vi "Main.vi"() -> ()   [LabVIEW 2013]
doc: "This template is for the Queued Message Handler design pattern.\n\nThe Event Handling Loop generates messages based on user interface actions.\n\nThe Message Handling Loop processes messages generated by the Event Handling Loop, or by other messages. The messages are string values, so new messages can be added easily to the Message Cases case structure in the Message Handling Loop. Each message cluster can also provide an optional value for Message Data, which is a variant that can be converted to whatever message-specific data is required."
uses:
  <vilib>/vision/Image Controls.llb/IMAQ Image.ctl
  Message Passing/MsgQ Loops enum.ctl
  Image Processing/Mask ROI FG Enum.ctl
  System Status/Status FG Enum.ctl
  Globals/Average Sector Data.vi
  controls/UI Data.ctl
  Message Queue/Message Queue.lvlib
  User Event - Stop/User Event - Stop.lvlib
  Image Processing/Image Processing.lvlib
  Common/State Machines/State Machine Lib.lvlib
  Message Passing/Main MsgQ.lvlib
  Common/GUI/GUI.lvlib
panel:
  out "Log Start (s)":dbl caption="Present (s)"
  in  "minutes to log":dbl=22.0
  out "Acq FIFO Timeout":bool
  out "Host DMA Timeout":bool
  in  "Log?":bool
  out "Log Input Signal":bool
  out "# of extracted frames":u32=1
  in  "Update Display?":bool=TRUE
  out "write time":dbl
  out "Frame Count":u16=1
  out "Frames Acquired":u32=11578
  in  "Disable Background Subtraction":bool
  out "FPGA Display Image":T1(plugin-control)
  out "Right Wingbeat Avg Graph":u8[](graph)=[71, 91, 86, 73, 55, 38, 22, 8, 3, 0, 0, 0, 0, 0, 0, 0]
  in  "Start Serial Server":bool=TRUE
  out "Left Wingbeat Avg Graph":u8[](graph)=[106, 114, 100, 76, 51, 28, 9, 0, 0, 0, 0, 0, 0, 0, 0, 0]
  in  "Stop Charts":bool
  in  "Wing ROIs":T2
  out "FPGA image info":T5={"Image Type"=0, "Unit"=enum."Undefined", "X Resolution"=1200, "Y Resolution"=788, "X Step"=1.0, "Y Step"=1.0, "Image Name"="Acquired"} {"Image Type" items=["Grayscale (U8)", "Grayscale (I16)", "Grayscale (SGL)", "Complex (CSG)", "RGB (U32)", "HSL (U32)", "RGB (U64)", "Grayscale (U16)"]}
  in  "Stream?":bool
  out "FPGA Image":T1
  in  "Test Visual Response":bool
  in  "Test FPGA":bool
  out "Status Update":string="09/25/2015 16:02:54.861 :  Camera Initialized\r"
  in  "Define Mask":bool
  in  "Acquire Image":bool
  in  "Stop":bool
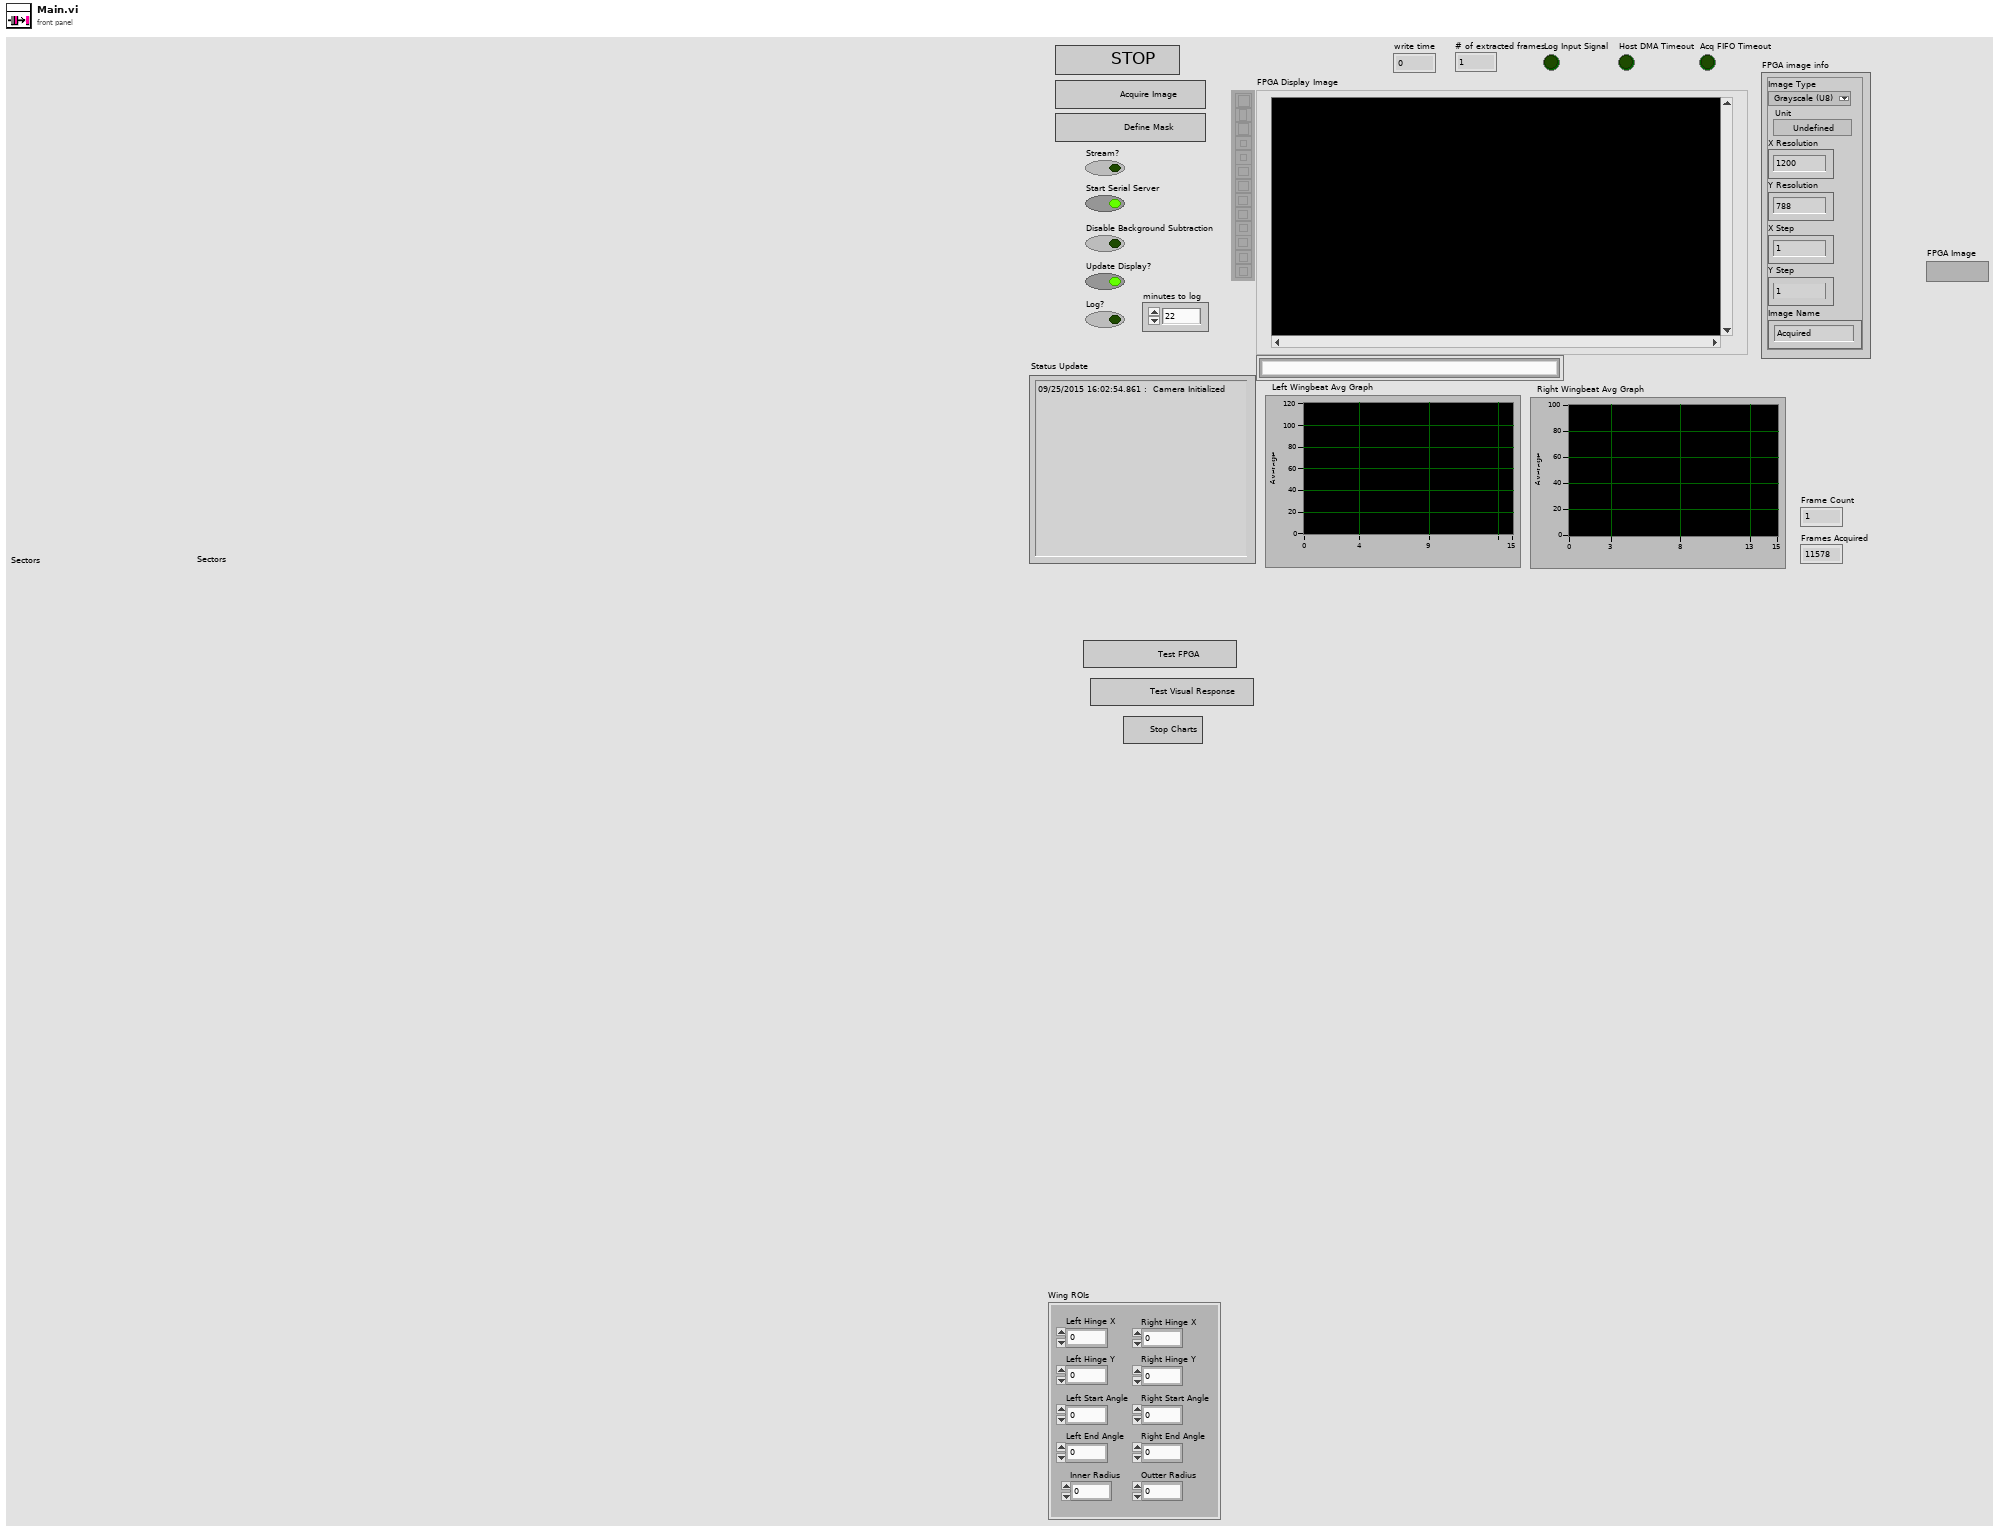
[diagram p1: front panel]
types:
  T1 = typedef "IMAQ Image.ctl" = refnum<image>
  T2 = cluster{"Left Hinge X":u16, "Left Hinge Y":u16, "Inner Radius":u16, "Outter Radius":u16, "Right Hinge X":u16, "Right Hinge Y":u16, "Right Start Angle":i16, "Right End Angle":i16, "Left Start Angle":i16, "Left End Angle":i16}
  T3 = typedef "Image Type" = u32
  T4 = typedef "Image Unit" = enum32{"Undefined", "Angström", "Micrometer", "Millimeter", "Centimeter", "Meter", "Kilometer", "Microinch", "Inch", "Feet", "Nautical miles", "Standard miles", "Steps"}
  T5 = cluster{"Image Type":T3, "Unit":T4, "X Resolution":i32, "Y Resolution":i32, "X Step":sgl, "Y Step":sgl, "Image Name":string}
  T6 = typedef "State Machine Lib.lvlib/STATE cluster.ctl" = cluster{"State":string, "Parameters":variant}
  T7 = typedef "Main MsgQ.lvlib/MsgQ Loops enum.ctl" = enum16{"User Interface", "Image Acq"}
  T8 = typedef "Mask ROI FG Enum.ctl" = enum16{"Read", "Write", "Enable Background", "Disable Background"}
  T9 = typedef "Status FG Enum.ctl" = enum16{"Reset", "Read", "Write"}
  T10 = typedef "Mask ROI Cluster.ctl" = cluster{"left annulus":T11, "right annulus":T11, "Threshold Range":cluster{"Lower value":dbl, "Upper value":dbl}, "[Avg BG]":u8[], "Number of Sectors":u8, "Left ROI":T12, "Right ROI":T12, "Left Start Angle Duty Cycle":fxp<+,8,0>, "Left End Angle Duty Cycle":fxp<+,8,0>, "Right End Angle Duty Cycle":fxp<+,8,0>, "Right Start Angle Duty Cycle":fxp<+,8,0>, "[Sector ROIs]":T12[], "Consecutive Sector Threshold":u8}
  T11 = typedef "IMAQ Circle" = cluster{"Center X":i32, "Center Y":i32, "Inner Radius":i32, "Outer Radius":i32, "Start Angle":dbl, "End Angle":dbl}
  T12 = typedef "ROI Descriptor" = cluster{"Global Rectangle":i32[], "Contours":cluster{"ID":enum32{"External", "Internal"}, "Type":u32, "Coordinates":i32[]}[]}
  T13 = typedef "UI Data.ctl" = cluster{"Boolean <Replace Me>":bool, "Initial Message":string, "Numeric <Replace Me>":dbl, "Acquire Image Ref":refnum<vi>, "Define Mask Ref":refnum<vi>, "Status Update Ref":refnum<vi>, "Stop Button Ref":refnum<vi>, "FPGA Image":T1, "Processed Image":T1, "Left Annulus":cluster{"Center X":i32, "Center Y":i32, "Inner Radius":i32, "Outer Radius":i32, "Start Angle":dbl, "End Angle":dbl}, "Right Annulus":cluster{"Center X":i32, "Center Y":i32, "Inner Radius":i32, "Outer Radius":i32, "Start Angle":dbl, "End Angle":dbl}}
  T14 = typedef "Message Queue.lvlib/All Message Queues.ctl" = cluster{"UI":refnum<queue>}
  T15 = cluster{"Center X":i32, "Center Y":i32, "Inner Radius":i32, "Outer Radius":i32, "Start Angle":dbl, "End Angle":dbl}
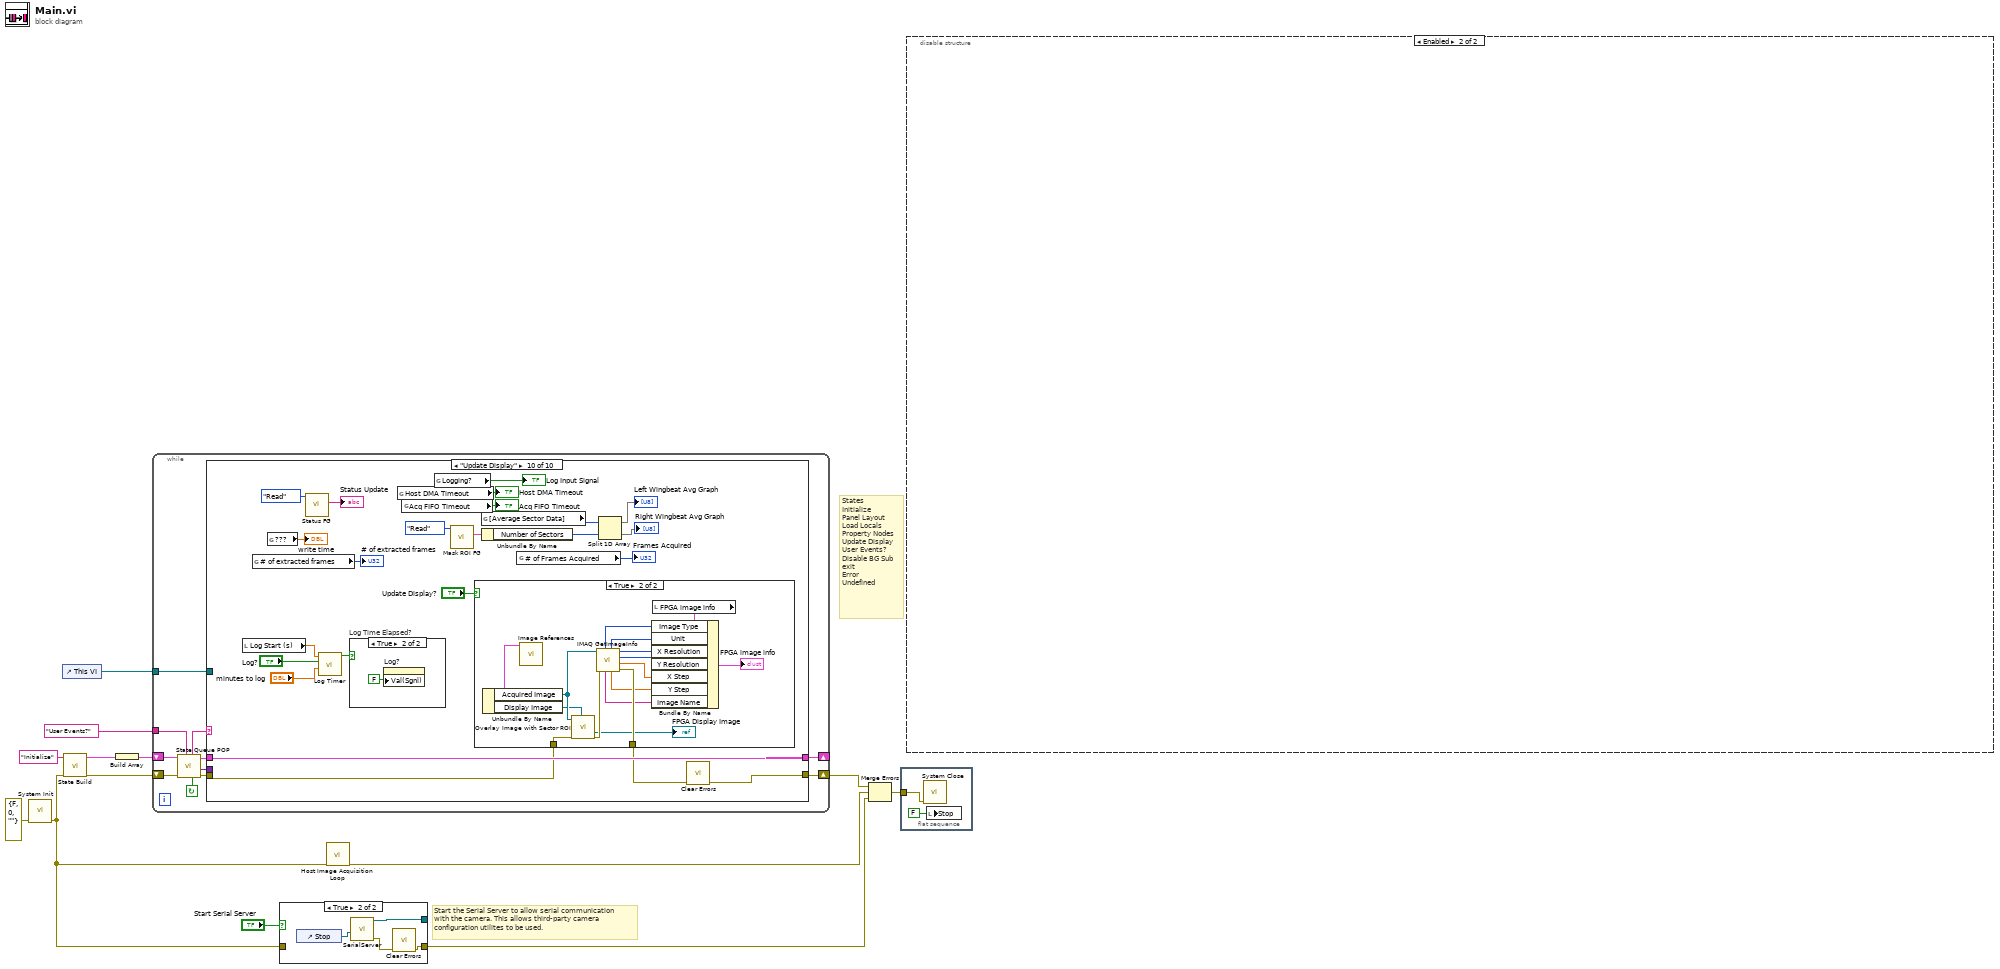
[diagram p0: block diagram]
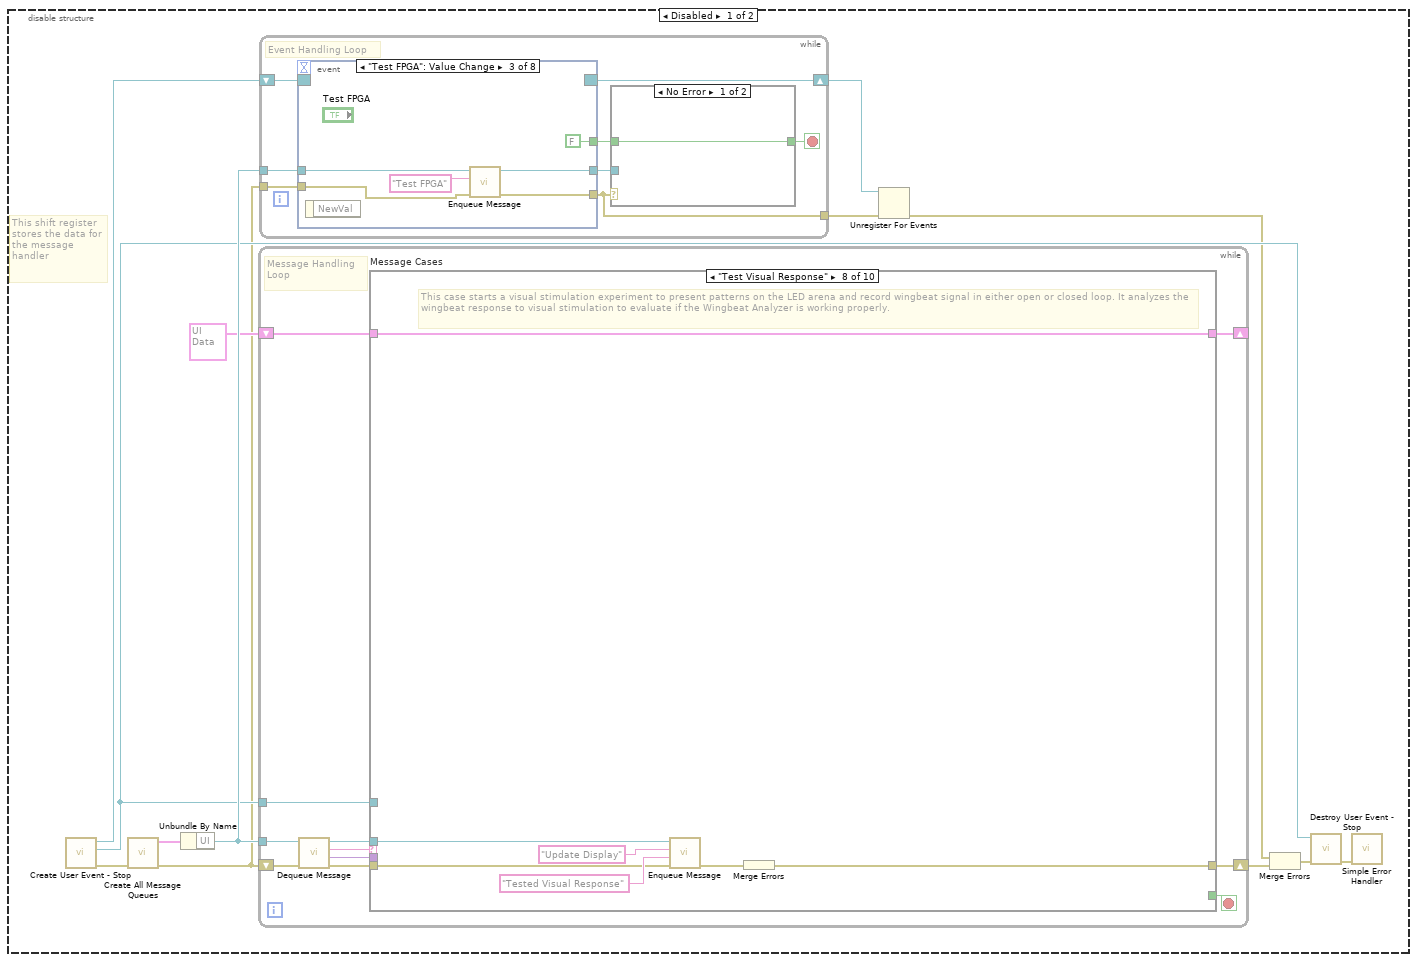
[diagram p3: hidden frame]
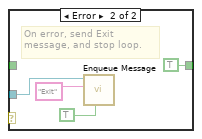
[diagram p4: hidden frame]
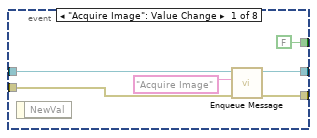
[diagram p5: hidden frame]
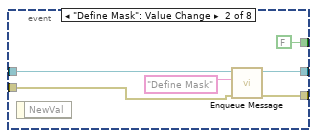
[diagram p6: hidden frame]
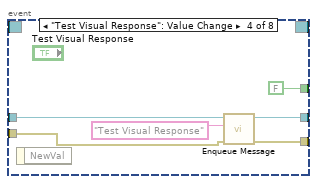
[diagram p7: hidden frame]
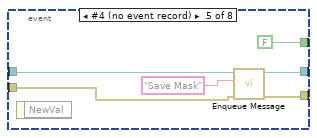
[diagram p8: hidden frame]
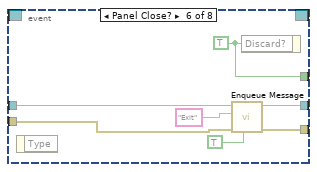
[diagram p9: hidden frame]
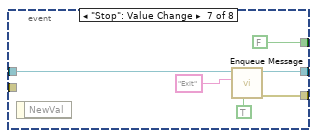
[diagram p10: hidden frame]
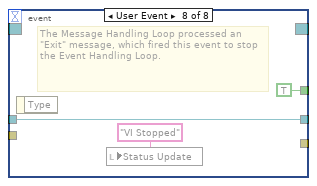
[diagram p11: hidden frame]
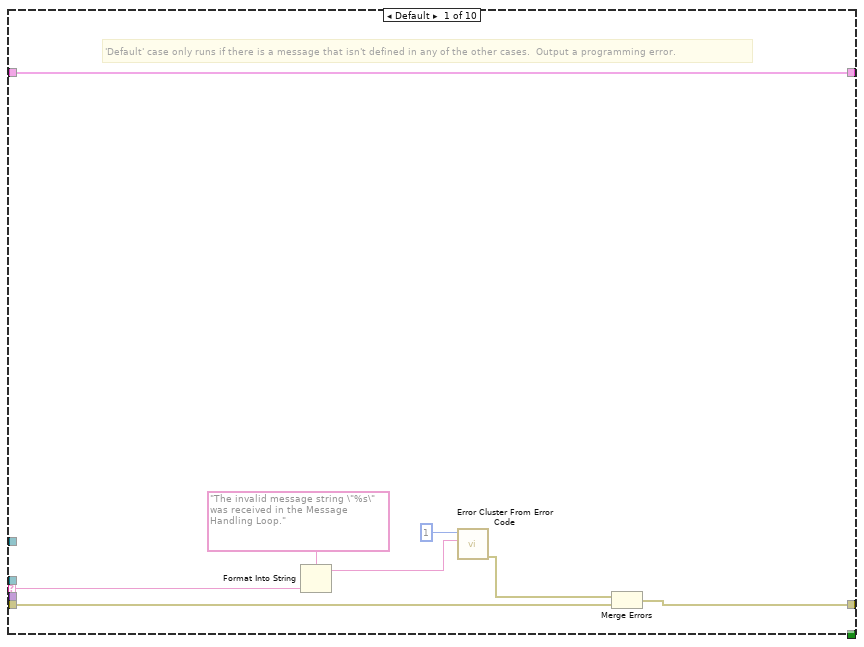
[diagram p12: hidden frame]
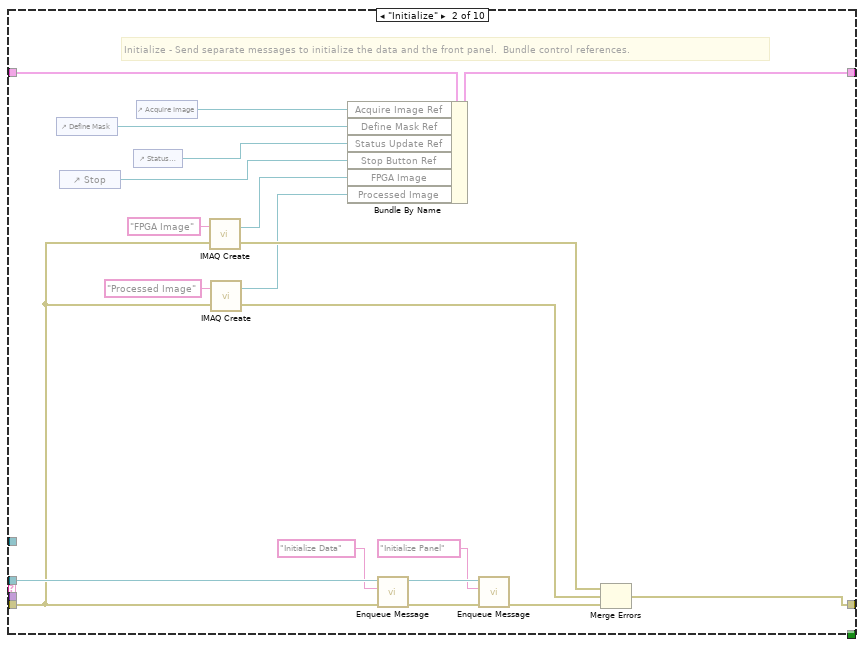
[diagram p13: hidden frame]
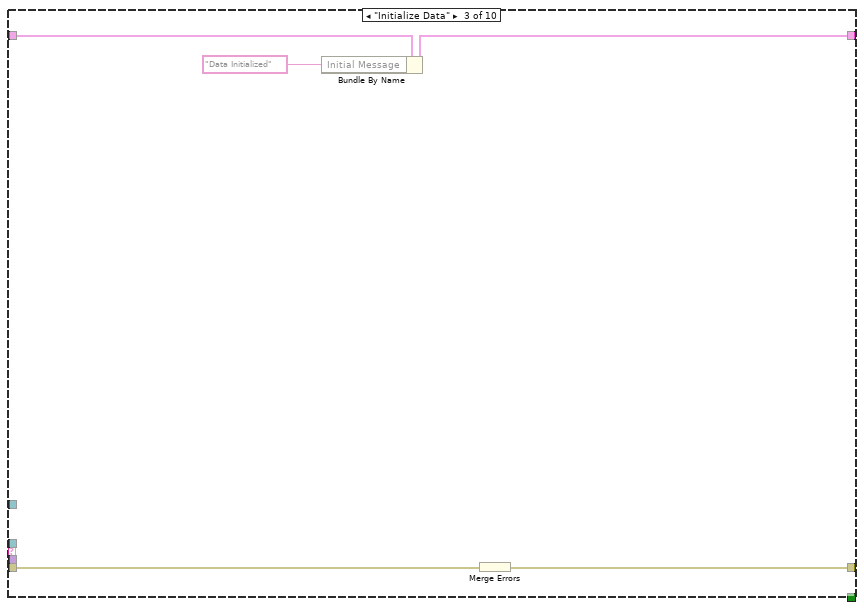
[diagram p14: hidden frame]
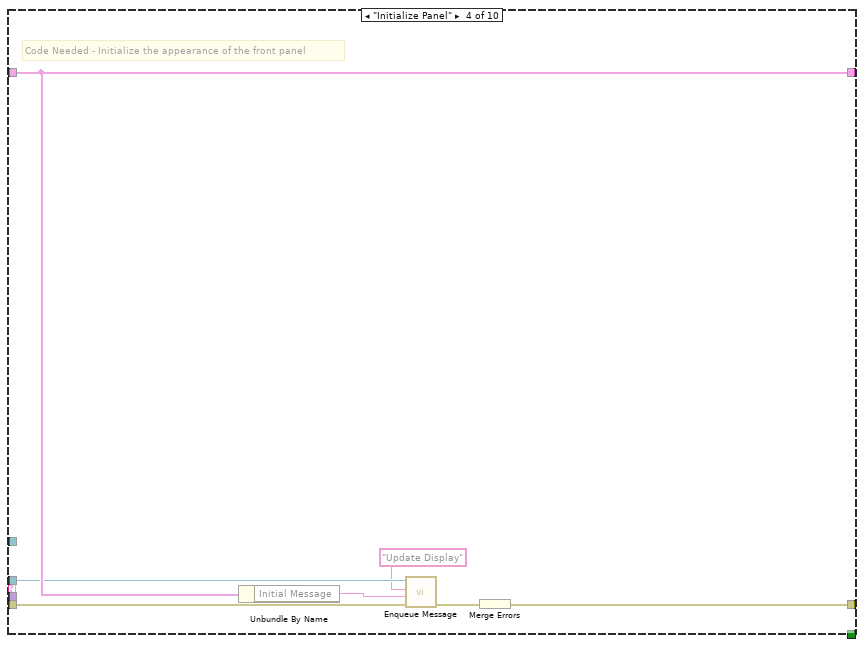
[diagram p15: hidden frame]
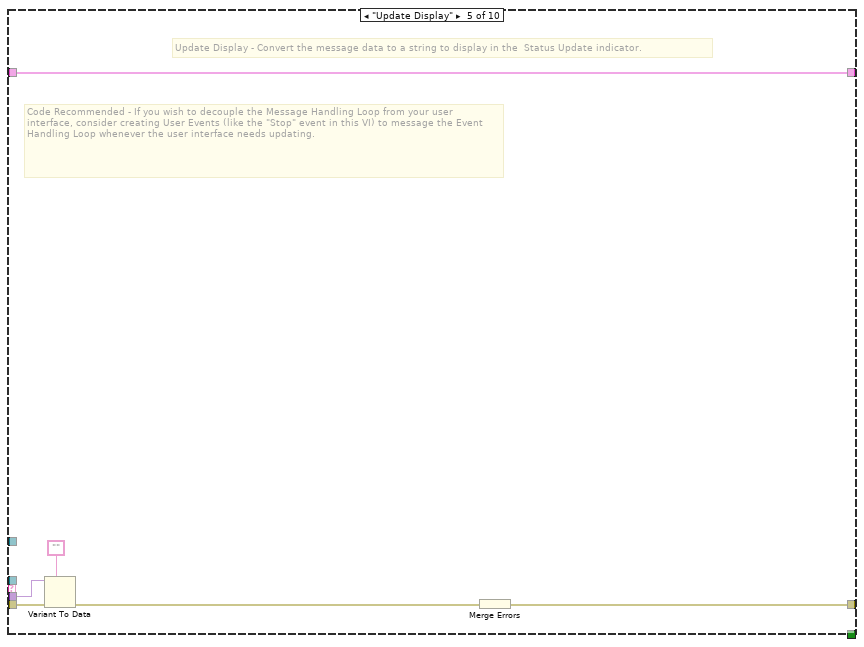
[diagram p16: hidden frame]
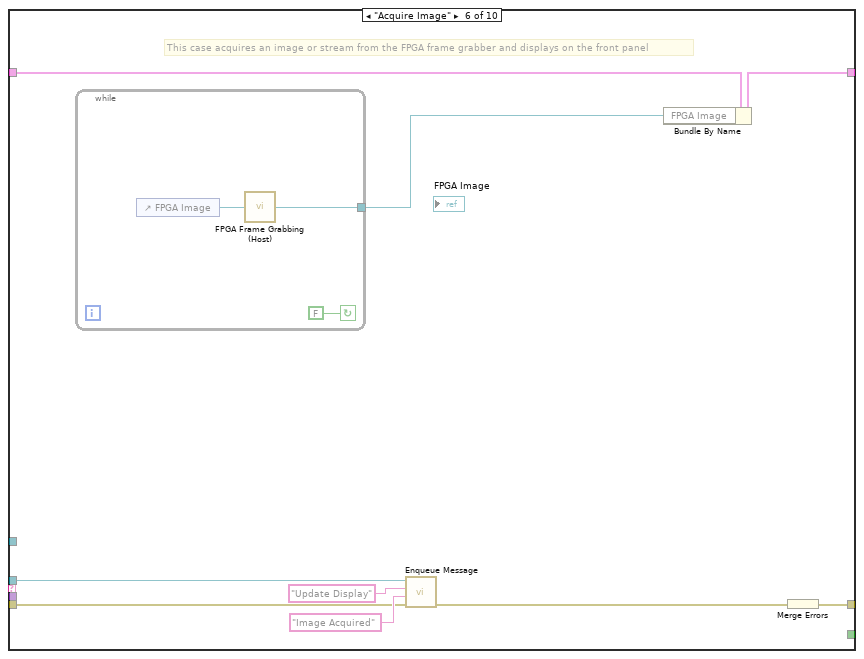
[diagram p17: hidden frame]
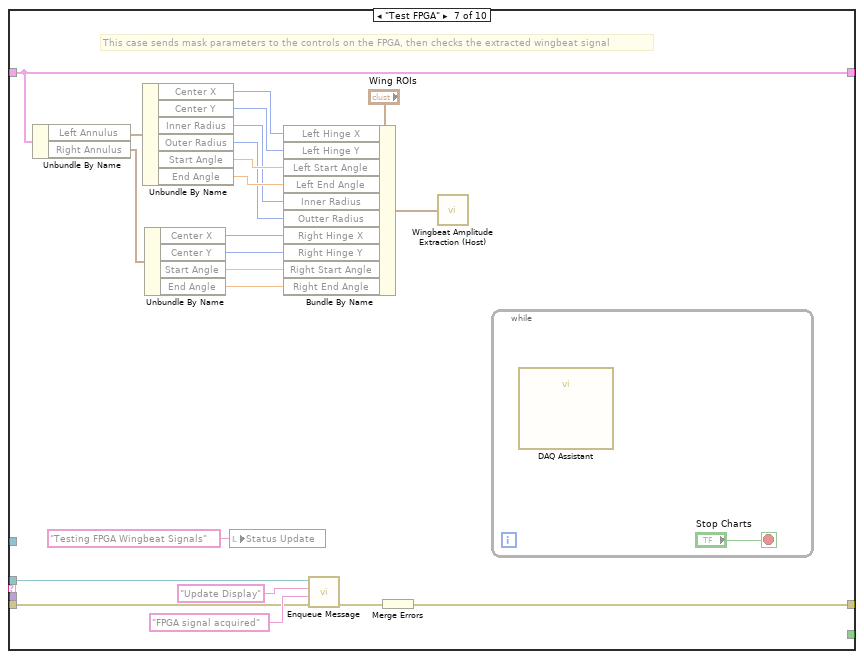
[diagram p18: hidden frame]
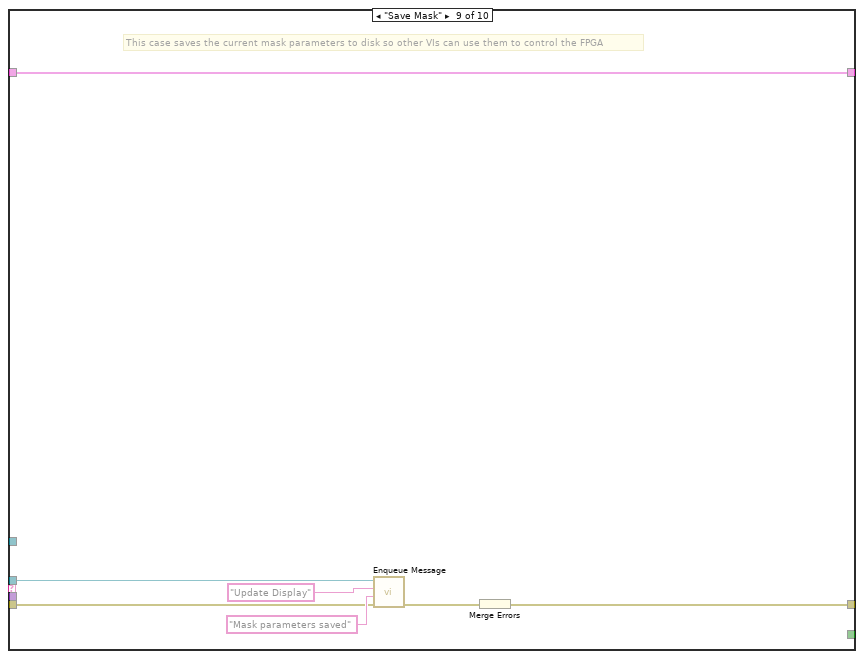
[diagram p19: hidden frame]
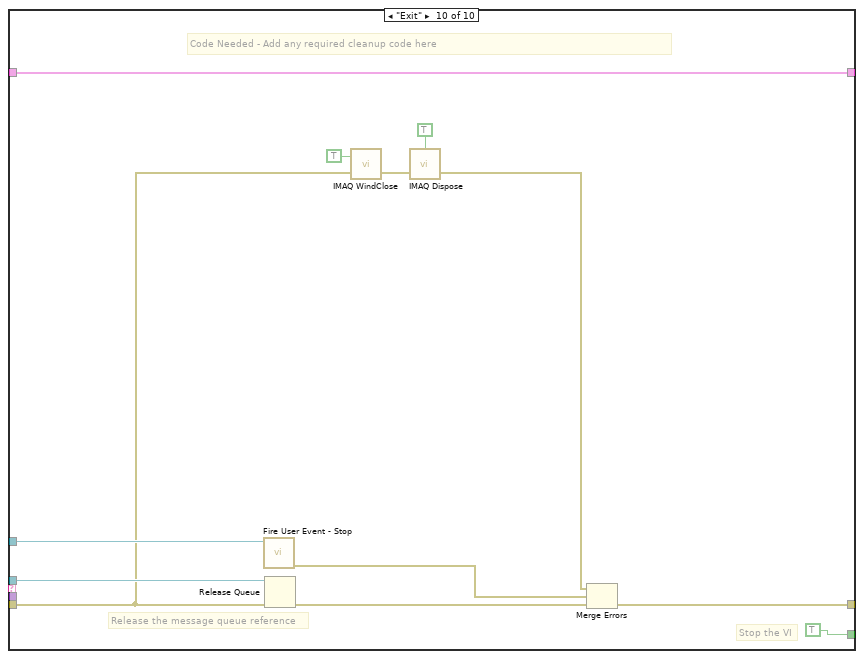
[diagram p20: hidden frame]
diagram:
  # "Start the Serial Server to allow serial communication\nwith the camera. This allows third-party camera\nconfiguration utilites to be used."
  # "States\nInitialize\nPanel Layout\nLoad Locals\nProperty Nodes\nUpdate Display\nUser Events?\nDisable BG Sub\nexit\nError\nUndefined"
  n1 = call "System Init.vi"("error in (no error)"=errorcluster {"status"=FALSE, "code"=0, "source"=""}) -> ("error out"=w12:errorcluster)  [unwired: 10 in]
  n2 = control-ref of="This VI"() -> (w6:refnum<vi>)
  n3 = call "State Build.vi"("error in (no error)"=w12, "State"="Initialize") -> ("error out"=w8:errorcluster, "State Out"=w10:T6)  [unwired: 8 in]
  n4 = Build Array(w10) -> (w9:T6[])
  n5 = while {
    shift-right: [w18] -> _
    shift-left: w9 -> [w24]
    shift-right: [w16] -> w5
    shift-left: w8 -> [w23]
    tunnel: "User Events?" ("State") -> [w21]
    tunnel: w6 -> [w19]
    stop <- w22 continue-if-true
    n6 = call "State Queue POP.vi"("Default state"=w21, "error in (no error)"=w23, "State que in"=w24) -> ("error out"=w15:errorcluster, "Parameters"=w14:variant, "State que out"=w17:T6[], "Not Exit?"=w22:bool, "State case out"=w20:string)  [unwired: 4 in]
    n7 = case shown="\"Update Display\"" w20 {
      tunnel: w19 -> [_ _ w35 _ _ _ _ _ _ _]
      tunnel: [w26 w27 w32 w41 w43 w48 w49 w66 w113 w137] -> w18
      tunnel: w17 -> [w26 w30 w32 w41 w43 w48 w49 w65 _ w137]
      tunnel: [w25 w28 w33 w36 w42 w46 w50 w64 w112 w136] -> w16
      tunnel: w15 -> [w25 w29 w34 w37 w42 w47 w61 w63 w114 w135]
      tunnel: w14 -> [_ _ _ _ _ _ w60 w62 _ _]
      frame Default {
      }
      frame "Initialize" {
        n8 = call "State Queue PUSH multiple states no parameters.vi"("States to queue"=string[] ["Panel Layout", "Load Locals", "Property Nodes", "Update Display"], "error in (no error)"=w29, "State que in"=w30) -> ("error out"=w28:errorcluster, "State que out"=w27:T6[])  [unwired: 7 in]
      }
      frame "Panel Layout" {
        # "Reset origin to 0,0"
        n9 = call "Reset all pane origins.vi"("error in (no error"=w34, "Vi Ref In"=w35) -> ("error out"=w33:errorcluster)  [unwired: 8 in, 1 out]
      }
      frame "Load Locals" {
        w40 = FALSE ("Stream?")
        n10 = call "Send MsgQ.vi"("error in (no error)"=w37, "Message String"="Close Save File" ("f"), "Send to MsgQ"=MsgQ_Loops_enum."Image Acq") -> ("error out"=w36:errorcluster)  [unwired: 8 in]
        n11 = local write "Stream?"(w40) -> ()
        n12 = local write "Disable Background Subtraction"(w40) -> ()
        n13 = local write "Log?"(w40) -> ()
      }
      frame "Property Nodes" {
      }
      frame "Define Mask" {
        n14 = call "Image References.vi"() -> ("Images"=w45:cluster{"Acquired Image":T1, "Display Image":T1})  [unwired: 10 in, 1 out]
        n15 = Unbundle By Name(w45) -> ("Acquired Image"=w44:T1)
        n16 = call "Define Mask.vi"("error in (no error)"=w47, "FPGA Image"=w44) -> ("error out"=w46:errorcluster)  [unwired: 9 in]
      }
      frame "Disable BG Sub" {
        n17 = Variant To Data(error in=w61, type=FALSE, Variant=w60) -> (data=w58:bool, error out=w55:errorcluster)
        n18 = Select(t=Mask_ROI_FG_Enum."Disable Background" ("Operation"), s=w58, f=Mask_ROI_FG_Enum."Enable Background" ("Operation")) -> (s? t:f=w54:T8)
        n19 = call "Mask ROI FG.vi"("error in (no error)"=w55, "Operation"=w54) -> ("error out"=w51:errorcluster)  [unwired: 8 in, 1 out]
        n20 = call "Send MsgQ.vi"("error in (no error)"=w51, "Message String"="Update Sector Parameters", "Send to MsgQ"=MsgQ_Loops_enum."Image Acq") -> ("error out"=w50:errorcluster)  [unwired: 8 in]
      }
      frame "User Events?" {
        n21 = event shown="[3] \"Log?\": Value Change" {
          selector: _ -> [_ _ _ _ _ _ _]
          dyn-events: _ -> [_ _ _ _ _ _ _]
          timeout: 200 -> [_ _ _ _ _ _ _]
          tunnel: [w69 w79 w83 w94 w98 w104 w107] -> w66
          tunnel: w65 -> [w70 w79 w83 w94 w100 w106 w110]
          tunnel: [w71 w76 w84 w92 w97 w103 w108] -> w64
          tunnel: w63 -> [w72 w77 w81 w93 w99 w105 w109]
          tunnel: w62 -> [_ _ _ _ _ _ _]
          event Timeout {
            n22 = event-data() -> ()  [unwired: 1 in, 3 out]
            n23 = call "State Queue PUSH.vi"("State case"="Update Display", "error in (no error)"=w72, "State que in"=w70) -> ("error out"=w71:errorcluster, "State que out"=w69:T6[])  [unwired: 7 in]
          }
          event "Acquire Image": Value Change {
            n24 = event-data() -> ()  [unwired: 1 in, 6 out]
            n25 = feedback #1(u16 0 ("Frame Count")) -> (w74:u16)
            n26 = call "Send MsgQ.vi"("error in (no error)"=w77, "Message String"="Acquire Single Image", "Send to MsgQ"=MsgQ_Loops_enum."Image Acq") -> ("error out"=w76:errorcluster)  [unwired: 8 in]
            n27 = Increment(x=w74) -> (x+1=w73:u16)
            "Frame Count" <- w73
            n28 = feedback-in #1(w73) -> ()
          }
          event "Stream?": Value Change {
            n29 = event-data() -> ("NewVal"=w82:bool)  [unwired: 1 in, 5 out]
            n30 = call "Send MsgQ.vi"("error in (no error)"=w81, "Data In"=w82, "Message String"="Stream Image", "Send to MsgQ"=MsgQ_Loops_enum."Image Acq") -> ("error out"=w84:errorcluster)  [unwired: 7 in]
          }
          event "Log?": Value Change {
            n31 = event-data() -> ("NewVal"=w87:bool)  [unwired: 1 in, 5 out]
            n32 = case shown="True" w87 {
              frame False {
              }
              frame True {
                n33 = call "Elapsed Time2"() -> ("Present (s)"=→"Log Start (s)":dbl)  [unwired: 12 in, 7 out]
              }
            }
            n34 = Select(t="Create Save File" ("Message String"), s=w87, f="Close Save File") -> (s? t:f=w89:string)
            n35 = call "Send MsgQ.vi"("error in (no error)"=w93, "Message String"=w89, "Send to MsgQ"=MsgQ_Loops_enum."Image Acq") -> ("error out"=w92:errorcluster)  [unwired: 8 in]
          }
          event "Define Mask": Value Change {
            n36 = event-data() -> ()  [unwired: 1 in, 6 out]
            n37 = call "State Queue PUSH.vi"("State case"="Define Mask", "error in (no error)"=w99, "State que in"=w100) -> ("error out"=w97:errorcluster, "State que out"=w98:T6[])  [unwired: 7 in]
          }
          event "Disable Background Subtraction": Value Change {
            n38 = event-data() -> ("NewVal"=w101:bool)  [unwired: 1 in, 5 out]
            n39 = call "State Queue PUSH.vi"("State case"="Disable BG Sub", "error in (no error)"=w105, "Parameters"=w101, "State que in"=w106) -> ("error out"=w103:errorcluster, "State que out"=w104:T6[])  [unwired: 6 in]
          }
          event "Stop": Value Change {
            n40 = event-data() -> ()  [unwired: 1 in, 6 out]
            n41 = call "State Queue PUSH.vi"("State case"="exit", "error in (no error)"=w109, "State que in"=w110) -> ("error out"=w108:errorcluster, "State que out"=w107:T6[])  [unwired: 7 in]
          }
        }
      }
      frame "exit" {
        n42 = call "Broadcast Exit.vi"("error in"=w114) -> ("error out"=w112:errorcluster)  [unwired: 10 in]
        n43 = call "Queue EXIT state.vi"() -> ("Exit State Q"=w113:T6[])  [unwired: 1 in]
      }
      frame "Update Display" {
        n44 = local read "Log Start (s)"() -> (w118:dbl)
        n45 = global read "Average Sector Data.vi" "# of extracted frames"() -> (→"# of extracted frames":u32)
        n46 = global read "Average Sector Data.vi" "???"() -> (→"write time":dbl)
        n47 = call "Status FG.vi"("Operation"=Status_FG_Enum."Read") -> ("Status Out"=→"Status Update":string)  [unwired: 9 in, 1 out]
        n48 = call "Log Timer.vi"("minutes to log"="minutes to log", "Log?"="Log?", "Log Start (s)"=w118) -> ("Time has Elapsed"=w115:bool)  [unwired: 8 in]
        n49 = case "Log Time Elapsed?" shown="True" w115 {
          frame False {
          }
          frame True {
            n50 = property on="Log?" class="Bool (strict)"("Val(Sgnl)"=FALSE ("Value (Signaling)")) -> ()  [unwired: 2 in, 2 out]
          }
        }
        n51 = global read "Average Sector Data.vi" "Host DMA Timeout"() -> (→"Host DMA Timeout":bool)
        n52 = global read "Average Sector Data.vi" "Acq FIFO Timeout"() -> (→"Acq FIFO Timeout":bool)
        n53 = global read "Average Sector Data.vi" "Logging?"() -> (→"Log Input Signal":bool)
        n54 = call "Mask ROI FG.vi"("Operation"=Mask_ROI_FG_Enum."Read") -> ("Mask ROI Out"=w130:T10)  [unwired: 9 in, 1 out]
        n55 = case shown="True" "Update Display?" {
          tunnel: w135 -> [w139 w155]
          tunnel: [w139 w154] -> w134
          frame False {
          }
          frame True {
            n56 = call "Image References.vi"() -> ("Images"=w143:cluster{"Acquired Image":T1, "Display Image":T1})  [unwired: 10 in, 1 out]
            n57 = Unbundle By Name(w143) -> ("Acquired Image"=w142:T1, "Display Image"=w141:T1)
            n58 = call "Overlay Image with Sector ROI.vi"("FPGA Display Image In"=w141, "error in"=w155, "FPGA Image"=w142) -> ("error out"=w144:errorcluster, "FPGA Display Image Out"=→"FPGA Display Image":T1)  [unwired: 7 in]
            n59 = call "IMAQ GetImageInfo"("error in (no error)"=w144, "Image"=w142) -> ("error out"=w154:errorcluster, "X Step"=w149:sgl, "Y Resolution"=w148:i32, "X Resolution"=w147:i32, "Y Step"=w150:sgl, "Unit"=w146:T4, "Image Name"=w151:string, "Image Type"=w145:T3)  [unwired: 2 in]
            n60 = local read "FPGA image info"() -> (w153:T5)
            n61 = Bundle By Name(cluster=w153, "Image Type"=w145, "Unit"=w146, "X Resolution"=w147, "Y Resolution"=w148, "X Step"=w149, "Y Step"=w150, "Image Name"=w151) -> (→"FPGA image info":T5)
          }
        }
        n62 = global read "Average Sector Data.vi" "[Average Sector Data]"() -> (w132:u8[])
        n63 = Unbundle By Name(w130) -> ("Number of Sectors"=w127:u8)
        n64 = global read "Average Sector Data.vi" "# of Frames Acquired"() -> (→"Frames Acquired":u32)
        n65 = Split 1D Array(array=w132, index=w127) -> (first subarray=→"Left Wingbeat Avg Graph":u8[], second subarray=→"Right Wingbeat Avg Graph":u8[])
        n66 = call <vilib>:"Clear Errors.vi"("error in (no error)"=w134) -> ("error out"=w136:errorcluster)  [unwired: 6 in]
      }
    }
  }
  n67 = case shown="True" "Start Serial Server" {
    tunnel: [_ w160] -> _
    tunnel: w12 -> [w156 _]
    tunnel: [w156 w158] -> w2
    frame False {
    }
    frame True {
      n68 = control-ref of="Stop"() -> (w159:refnum<vi>)
      n69 = call "SerialServer.vi"("Stop Refnum"=w159) -> ("error out"=w157:errorcluster, "FPGA VI Reference Out"=w160:refnum<k20>)  [unwired: 5 in]
      n70 = call <vilib>:"Clear Errors.vi"("error in (no error)"=w157) -> ("error out"=w158:errorcluster)  [unwired: 6 in]
    }
  }
  n71 = call "Host Image Acquisition Loop.vi"("error in"=w12) -> ("error out"=w4:errorcluster)  [unwired: 10 in]
  n72 = Merge Errors(w5, w4, w2) -> (w3:errorcluster)
  n73 = flat-sequence {
    tunnel: w3 -> [w162]
    frame #0 {
      n74 = call "System Close.vi"("error in (no error)"=w162) -> ()  [unwired: 10 in, 1 out]
      n75 = local write "Stop"(FALSE ("Stop")) -> ()
    }
  }
  n76 = disable-structure shown="Enabled" {
    frame Disabled {
      # "This shift register\nstores the data for the message handler"
      n77 = call "Create User Event - Stop.vi"() -> ("error out"=w171:errorcluster, "User Event - Stop"=w168:refnum<user-event>, "Stop Event Registration Refnum"=w172:refnum<event-registration>)  [unwired: 9 in]
      n78 = call "Create All Message Queues.vi"("error in (no error)"=w171) -> ("error out"=w163:errorcluster, "Message Queues out"=w175:T14)  [unwired: 9 in]
      n79 = Unbundle By Name(w175) -> ("UI"=w173:refnum<queue>)
      n80 = while {
        tunnel: w173 -> [w235]
        shift-right: [w244] -> _
        shift-left: T13 {"Boolean <Replace Me>"=TRUE, "Initial Message"="", "Numeric <Replace Me>"=0.0, "Acquire Image Ref"=refnum, "Define Mask Ref"=refnum, "Status Update Ref"=refnum, "Stop Button Ref"=refnum, "FPGA Image"=refnum, "Processed Image"=refnum, "Left Annulus"={"Center X"=0, "Center Y"=0, "Inner Radius"=0, "Outer Radius"=0, "Start Angle"=0.0, "End Angle"=0.0}, "Right Annulus"={"Center X"=0, "Center Y"=0, "Inner Radius"=0, "Outer Radius"=0, "Start Angle"=0.0, "End Angle"=0.0}} ("Data Cluster") -> [w245]
        tunnel: w168 -> [w241]
        shift-right: [w242] -> w174
        shift-left: w163 -> [w240]
        stop <- w243 stop-if-true
        # "Message Handling Loop"
        n81 = call "Dequeue Message.vi"("error in (no error)"=w240, "Message Queue"=w235) -> ("error out"=w239:errorcluster, "Message Data"=w237:variant, "Message"=w238:string, "dup Message Queue"=w236:refnum<queue>)  [unwired: 6 in]
        n82 = case "Message Cases" shown="\"Test Visual Response\"" w238 {
          selector: w238 -> [w251 _ _ _ _ _ _ _ _ _]
          tunnel: w236 -> [_ w271 _ w282 _ w299 w322 w330 w338 w354]
          tunnel: w239 -> [w248 w256 w278 w283 w290 w294 w323 w331 w336 w343]
          tunnel: [w246 w258 w274 w284 w291 w301 w321 w329 w341 w350] -> w242
          tunnel: w245 -> [w253 w268 w277 w285 w292 w296 w320 w335 w342 w353]
          tunnel: [w253 w267 w276 w285 w292 w295 w320 w335 w342 w353] -> w244
          tunnel: [_ _ _ _ _ _ _ _ _ TRUE] -> w243
          tunnel: w237 -> [_ _ _ _ w289 _ _ _ _ _]
          tunnel: w241 -> [_ _ _ _ _ _ _ _ _ w349]
          frame Default {
            # "'Default' case only runs if there is a message that isn't defined in any of the other cases.  Output a programming error."
            n83 = Format Into String(format string="The invalid message string \"%s\" was received in the Message Handling Loop." ("Unknown Message Error Text"), w251) -> (resulting string=w249:string)  [unwired: 2 in, 1 out]
            n84 = call <vilib>:"Error Cluster From Error Code.vi"("error message (\"\")"=w249, "error code (0)"=1) -> ("error out"=w247:errorcluster)  [unwired: 7 in]
            n85 = Merge Errors(w247, w248) -> (w246:errorcluster)
          }
          frame "Initialize" {
            # "Initialize - Send separate messages to initialize the data and the front panel.  Bundle control references."
            n86 = control-ref of="Define Mask"() -> (w265:refnum<vi>)
            n87 = control-ref of="Stop"() -> (w263:refnum<vi>)
            n88 = control-ref of="Status Update"() -> (w264:refnum<vi>)
            n89 = control-ref of="Acquire Image"() -> (w266:refnum<vi>)
            n90 = call "IMAQ Create"("Image Name"="FPGA Image", "error in (no error)"=w256) -> ("New Image"=w261:T1, "error out"=w257:errorcluster)  [unwired: 3 in]
            n91 = call "IMAQ Create"("Image Name"="Processed Image", "error in (no error)"=w256) -> ("New Image"=w254:T1, "error out"=w255:errorcluster)  [unwired: 3 in]
            n92 = Bundle By Name(cluster=w268, "Acquire Image Ref"=w266, "Define Mask Ref"=w265, "Status Update Ref"=w264, "Stop Button Ref"=w263, "FPGA Image"=w261, "Processed Image"=w254) -> (w267:T13)
            n93 = call "Enqueue Message.vi"("error in (no error)"=w256, "Message"="Initialize Data", "Message Queue"=w271) -> ("error out"=w273:errorcluster, "dup Message Queue"=w272:refnum<queue>)  [unwired: 7 in]
            n94 = call "Enqueue Message.vi"("error in (no error)"=w273, "Message"="Initialize Panel", "Message Queue"=w272) -> ("error out"=w259:errorcluster)  [unwired: 7 in, 1 out]
            n95 = Merge Errors(w257, w255, w259) -> (w258:errorcluster)
          }
          frame "Initialize Data" {
            n96 = Bundle By Name(cluster=w277, "Initial Message"="Data Initialized") -> (w276:T13)
            n97 = Merge Errors(w278) -> (w274:errorcluster)
          }
          frame "Initialize Panel" {
            # "Code Needed - Initialize the appearance of the front panel"
            n98 = Unbundle By Name(w285) -> ("Initial Message"=w279:string)
            n99 = call "Enqueue Message.vi"("error in (no error)"=w283, "Message Data"=w279, "Message"="Update Display", "Message Queue"=w282) -> ("error out"=w281:errorcluster)  [unwired: 6 in, 1 out]
            n100 = Merge Errors(w281) -> (w284:errorcluster)
          }
          frame "Update Display" {
            # "Code Recommended - If you wish to decouple the Message Handling Loop from your user interface, consider creating User Events (like the \"Stop\" event in this VI) to message the Event Handling Loop whenever the user interface needs updating."
            # "Update Display - Convert the message data to a string to display in the  Status Update indicator."
            n101 = Variant To Data(error in=w290, type="", Variant=w289) -> (data=w286:string, error out=w287:errorcluster)
            n102 = Merge Errors(w287) -> (w291:errorcluster)
          }
          frame "Acquire Image" {
            # "This case acquires an image or stream from the FPGA frame grabber and displays on the front panel"
            n103 = while {
              tunnel: [w304] -> w293
              stop <- FALSE continue-if-true
              n104 = control-ref of="FPGA Image"() -> (w303:refnum<vi>)
              n105 = call "FPGA Frame Grabbing (Host).vi"("Ctl Refnum"=w303) -> ("Image"=w304:T1)
            }
            n106 = call "Enqueue Message.vi"("error in (no error)"=w294, "Message Data"="Image Acquired" ("\"Do Something\" button pressed"), "Message"="Update Display", "Message Queue"=w299) -> ("error out"=w300:errorcluster)  [unwired: 6 in, 1 out]
            n107 = Bundle By Name(cluster=w296, "FPGA Image"=w293) -> (w295:T13)
            n108 = Merge Errors(w300) -> (w301:errorcluster)
          }
          frame "Test FPGA" {
            # "This case sends mask parameters to the controls on the FPGA, then checks the extracted wingbeat signal"
            n109 = Unbundle By Name(w320) -> ("Left Annulus"=w319:T15, "Right Annulus"=w318:T15)
            n110 = Unbundle By Name(w319) -> ("Center X"=w316:i32, "Center Y"=w315:i32, "Inner Radius"=w312:i32, "Outer Radius"=w311:i32, "Start Angle"=w314:dbl, "End Angle"=w313:dbl)
            n111 = Unbundle By Name(w318) -> ("Center X"=w310:i32, "Center Y"=w309:i32, "Start Angle"=w308:dbl, "End Angle"=w307:dbl)
            n112 = local write "Status Update"("Testing FPGA Wingbeat Signals" ("Status Update")) -> ()
            n113 = Bundle By Name(cluster="Wing ROIs", "Left Hinge X"=w316, "Left Hinge Y"=w315, "Left Start Angle"=w314, "Left End Angle"=w313, "Inner Radius"=w312, "Outter Radius"=w311, "Right Hinge X"=w310, "Right Hinge Y"=w309, "Right Start Angle"=w308, "Right End Angle"=w307) -> (w306:T2)
            n114 = call "Enqueue Message.vi"("error in (no error)"=w323, "Message Data"="FPGA signal acquired" ("\"Do Something\" button pressed"), "Message"="Update Display", "Message Queue"=w322) -> ("error out"=w326:errorcluster)  [unwired: 6 in, 1 out]
            n115 = Merge Errors(w326) -> (w321:errorcluster)
            n116 = call "Wingbeat Amplitude Extraction (Host).vi"("Wing ROIs"=w306) -> ()  [unwired: 1 in]
            n117 = while {
              stop <- "Stop Charts" stop-if-true
              n118 = call "DAQ Assistant"() -> ("data"=w327:dynamicdata)  [unwired: 17 in, 2 out]
            }
          }
          frame "Test Visual Response" {
            # "This case starts a visual stimulation experiment to present patterns on the LED arena and record wingbeat signal in either open or closed loop. It analyzes the wingbeat response to visual stimulation to evaluate if the Wingbeat Analyzer is working properly."
            n119 = call "Enqueue Message.vi"("error in (no error)"=w331, "Message Data"="Tested Visual Response" ("\"Do Something\" button pressed"), "Message"="Update Display", "Message Queue"=w330) -> ("error out"=w334:errorcluster)  [unwired: 6 in, 1 out]
            n120 = Merge Errors(w334) -> (w329:errorcluster)
          }
          frame "Save Mask" {
            # "This case saves the current mask parameters to disk so other VIs can use them to control the FPGA"
            n121 = call "Enqueue Message.vi"("error in (no error)"=w336, "Message Data"="Mask parameters saved" ("\"Do Something Else\" button pressed"), "Message"="Update Display", "Message Queue"=w338) -> ("error out"=w337:errorcluster)  [unwired: 6 in, 1 out]
            n122 = Merge Errors(w337) -> (w341:errorcluster)
          }
          frame "Exit" {
            # "Stop the VI"
            # "Release the message queue reference"
            # "Code Needed - Add any required cleanup code here"
            n123 = call "Fire User Event - Stop.vi"("User Event - Stop"=w349) -> ("error out"=w348:errorcluster)  [unwired: 10 in]
            n124 = Release Queue(queue=w354, error in (no error)=w343) -> (error out=w351:errorcluster)  [unwired: 1 in, 2 out]
            n125 = call "IMAQ WindClose"("Close All Windows (False)"=TRUE, "error in (no error)"=w343) -> ("error out"=w345:errorcluster)  [unwired: 4 in]
            n126 = call "IMAQ Dispose"("All Images? (No)"=TRUE, "error in (no error)"=w345) -> ("error out"=w344:errorcluster)  [unwired: 4 in]
            n127 = Merge Errors(w344, w348, w351) -> (w350:errorcluster)
          }
        }
      }
      n128 = while {
        tunnel: w173 -> [w183]
        tunnel: [w179] -> w166
        shift-right: [w177] -> w165
        shift-left: w172 -> [w178]
        tunnel: w163 -> [w176]
        stop <- w181 stop-if-true
        # "Event Handling Loop"
        n129 = event shown="[2] \"Test FPGA\": Value Change" {
          selector: w178 -> [_ _ _ _ _ _ _ _]
          dyn-events: [_ _ _ _ _ _ _ _] -> w177
          timeout: _ -> [_ _ _ _ _ _ _ _]
          tunnel: [FALSE ("Discard?") FALSE ("Discard?") FALSE ("Discard?") FALSE ("Discard?") FALSE ("Discard?") w225 FALSE ("Discard?") TRUE ("Discard?")] -> w182
          tunnel: w183 -> [w194 w200 w206 w211 w216 w224 w231 w234]
          tunnel: [w193 w198 w203 w208 w213 w223 w230 _] -> w179
          tunnel: [w192 w199 w202 w210 w215 w222 w228 w234] -> w180
          tunnel: w176 -> [w190 w196 w204 w207 w214 w219 _ _]
          event "Acquire Image": Value Change {
            n130 = event-data() -> ()  [unwired: 1 in, 1 out]
            n131 = call "Enqueue Message.vi"("error in (no error)"=w190, "Message"="Acquire Image", "Message Queue"=w194) -> ("error out"=w193:errorcluster, "dup Message Queue"=w192:refnum<queue>)  [unwired: 7 in]
          }
          event "Define Mask": Value Change {
            n132 = event-data() -> ()  [unwired: 1 in, 1 out]
            n133 = call "Enqueue Message.vi"("error in (no error)"=w196, "Message"="Define Mask", "Message Queue"=w200) -> ("error out"=w198:errorcluster, "dup Message Queue"=w199:refnum<queue>)  [unwired: 7 in]
          }
          event "Test FPGA": Value Change {
            n134 = event-data() -> ()  [unwired: 1 in, 1 out]
            n135 = call "Enqueue Message.vi"("error in (no error)"=w204, "Message"="Test FPGA", "Message Queue"=w206) -> ("error out"=w203:errorcluster, "dup Message Queue"=w202:refnum<queue>)  [unwired: 7 in]
          }
          event "Test Visual Response": Value Change {
            n136 = event-data() -> ()  [unwired: 1 in, 1 out]
            n137 = call "Enqueue Message.vi"("error in (no error)"=w207, "Message"="Test Visual Response", "Message Queue"=w211) -> ("error out"=w208:errorcluster, "dup Message Queue"=w210:refnum<queue>)  [unwired: 7 in]
          }
          event #4 (no event record) {
            n138 = event-data() -> ()  [unwired: 1 in, 1 out]
            n139 = call "Enqueue Message.vi"("error in (no error)"=w214, "Message"="Save Mask", "Message Queue"=w216) -> ("error out"=w213:errorcluster, "dup Message Queue"=w215:refnum<queue>)  [unwired: 7 in]
          }
          event Panel Close? {
            w225 = TRUE ("Discard?")
            n140 = event-data() -> ()  [unwired: 1 in, 1 out]
            n141 = call "Enqueue Message.vi"("Priority Message? (F)"=TRUE, "error in (no error)"=w219, "Message"="Exit", "Message Queue"=w224) -> ("error out"=w223:errorcluster, "dup Message Queue"=w222:refnum<queue>)  [unwired: 6 in]
            n142 = event-data("Discard?"=w225) -> ()  [unwired: 1 in, 1 out]
          }
          event "Stop": Value Change {
            n143 = event-data() -> ()  [unwired: 1 in, 1 out]
            n144 = call "Enqueue Message.vi"("Priority Message? (F)"=TRUE, "Message"="Exit", "Message Queue"=w231) -> ("error out"=w230:errorcluster, "dup Message Queue"=w228:refnum<queue>)  [unwired: 7 in]
          }
          event User Event {
            # "The Message Handling Loop processed an \"Exit\" message, which fired this event to stop the Event Handling Loop."
            n145 = event-data() -> ()  [unwired: 1 in, 1 out]
            n146 = local write "Status Update"("VI Stopped" ("VI Stopped")) -> ()
          }
        }
        n147 = case shown="No Error" w179 {
          tunnel: [w184 TRUE ("Discard?")] -> w181
          tunnel: w182 -> [w184 _]
          tunnel: w180 -> [_ w187]
          frame No Error {
          }
          frame Error {
            # "On error, send Exit message, and stop loop."
            n148 = call "Enqueue Message.vi"("Priority Message? (F)"=TRUE, "Message"="Exit", "Message Queue"=w187) -> ()  [unwired: 7 in, 2 out]
          }
        }
      }
      n149 = Unregister For Events(event registration refnum=w165, error in=w166) -> (error out=w167:errorcluster)
      n150 = Merge Errors(w167, w174) -> (w169:errorcluster)
      n151 = call "Destroy User Event - Stop.vi"("error in (no error)"=w169, "User Event - Stop"=w168) -> ("error out"=w170:errorcluster)  [unwired: 9 in]
      n152 = call <vilib>:"Simple Error Handler.vi"("error in (no error)"=w170) -> ()  [unwired: 4 in, 5 out]
    }
    frame Enabled {
    }
  }
